vi "Close pre-empt.vi"(8 "error in (no error)":errorcluster, 11 "_Popup in":refnum<class "Popup.lvclass">) -> (0 "error out":errorcluster)   [LabVIEW 2021, in "Pop-Up.lvlib" / "Popup.lvclass"]
doc: "get the pre-emptible notifier reference\n\n<b>Code Developed By:</b>\nTechnology Service Corporation\n1983 S Liberty Drive\nBloomington, IN 47403\nPhone: 812 558-7100\nwww.tsc.com/atcs"
uses:
  Popup.lvclass
  Popup.lvclass/Popup.ctl
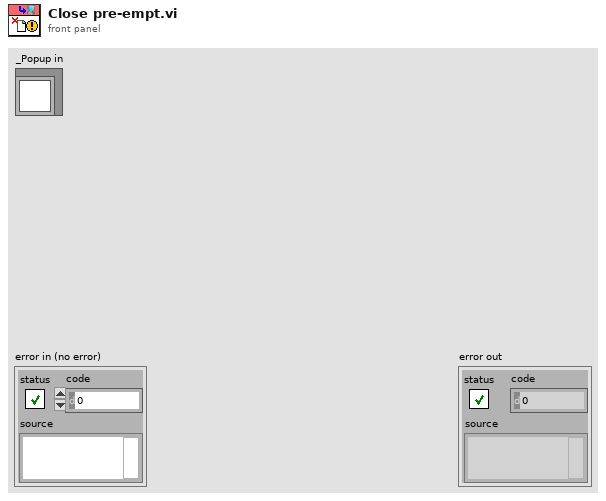
[diagram p1: front panel]
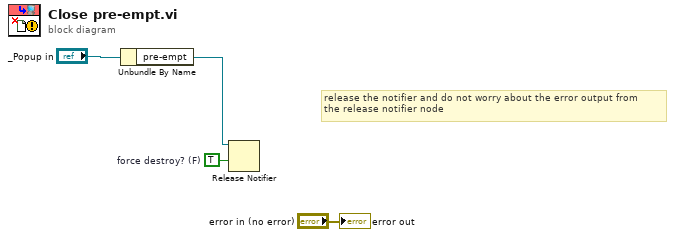
[diagram p0: block diagram]
diagram:
  w1 = TRUE  # force destroy? (F)
  # "release the notifier and do not worry about the error output from\nthe release notifier node"
  n1 = Unbundle By Name("_Popup in") -> ("pre-empt"=w2:refnum<notifier>)
  n2 = Release Notifier(notifier=w2, force destroy? (F)=w1) -> ()  [unwired: 1 in, 3 out]
  "error out" <- "error in (no error)"
